vi "GetLogFilePath.vi"(3 "Server name":string) -> (0 "LogFolder":path, 1 "LogPath":path)   [LabVIEW 2015]
doc: "Gets the path of a log file"
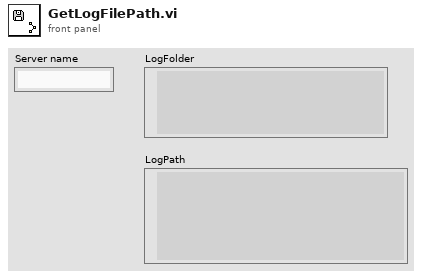
[diagram p1: front panel]
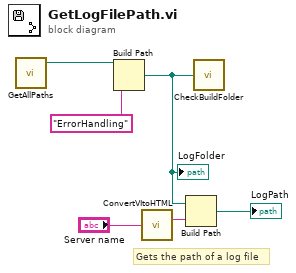
[diagram p0: block diagram]
diagram:
  # "Gets the path of a log file"
  n1 = call "GetAllPaths.vi"() -> ("User Documents"=w1:path)  [unwired: 1 in, 2 out]
  n2 = Build Path(base path=w1, name or relative path="ErrorHandling") -> (appended path=w4:path)
  "LogFolder" <- w4
  n3 = call "ConvertVItoHTML.vi"("vi name"="Server name") -> ("Htm log name"=w2:string)  [unwired: 1 out]
  n4 = Build Path(base path=w4, name or relative path=w2) -> (appended path=→"LogPath":path)
  n5 = call "CheckBuildFolder.vi"("appended path"=w4) -> ()  [unwired: 1 in]
